vi "Strip visual scanner brackets.vi"(8 "error in (no error)":errorcluster, 11 "Work order scan":string) -> (0 "error out":errorcluster, 3 "result string":string)   [LabVIEW 2013]
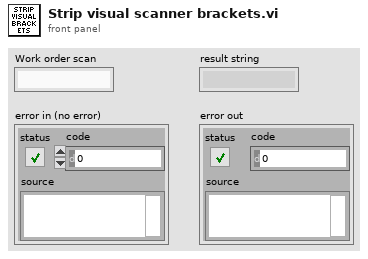
[diagram p1: front panel]
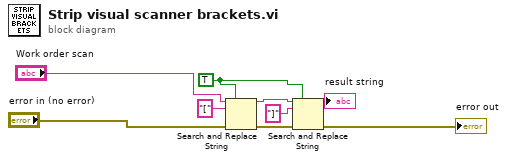
[diagram p0: block diagram]
diagram:
  w6 = TRUE ("replace all? (F)")
  n1 = Search and Replace String(replace all?=w6, input string="Work order scan", search string="[" ("regular expression"), error in="error in (no error)") -> (result string=w3:string, error out=w5:errorcluster)  [unwired: 4 in, 2 out]
  n2 = Search and Replace String(replace all?=w6, input string=w3, search string="]", error in=w5) -> (result string=→"result string":string, error out=→"error out":errorcluster)  [unwired: 4 in, 2 out]
